vi "Save-Defaults.vi"(8 "error in (no error)":errorcluster, 9 "VI path":path, 11 "configuration file path":path) -> (0 "error out":errorcluster)   [LabVIEW 2020, in "Save-Load-Defaults.lvlib"]
doc: "This VI saves the controls of the VI specified in VI path to settings.dat using the Configuration File VIs."
uses:
  Save-Load-Defaults.lvlib
  <vilib>/Utility/config.llb/Write Key (String).vi
  <vilib>/Utility/config.llb/NI_LVConfig.lvlib
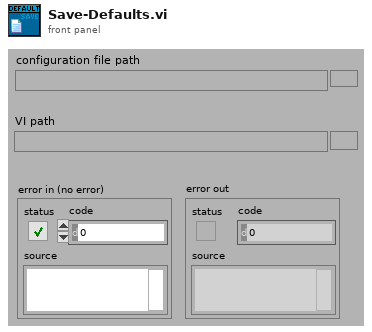
[diagram p1: front panel]
types:
  T1 = typedef "NI_LVConfig.lvlib/Config Data RefNum.ctl" = refnum<k1>
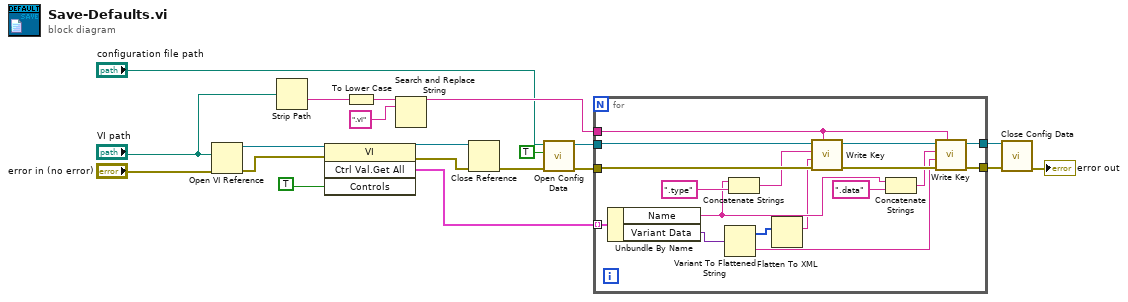
[diagram p0: block diagram]
diagram:
  n1 = Open VI Reference(vi path="VI path", error in (no error)="error in (no error)") -> (vi reference=w4:refnum<vi>, error out=w6:errorcluster)  [unwired: 4 in]
  n2 = Strip Path(path="VI path") -> (name=w19:string)  [unwired: 1 out]
  n3 = invoke class="VI" method="Ctrl Val.Get All"(reference=w4, error in=w6, "Controls"=TRUE ("controls")) -> (reference out=w8:refnum<vi>, error out=w9:errorcluster, "Get All Control Values Variant"=w7:cluster{"Name":string, "Variant Data":variant}[])  [unwired: 1 in, 1 out]
  n4 = To Lower Case(string=w19) -> (all lower case string=w20:string)
  n5 = Search and Replace String(input string=w20, search string=".vi") -> (result string=w18:string)  [unwired: 6 in, 3 out]
  n6 = Close Reference(reference=w8, error in (no error)=w9) -> (error out=w14:errorcluster)
  n7 = call <vilib>:"Open Config Data.vi"("error in (no error)"=w14, "create file if necessary (T)"=TRUE, "configuration file path"="configuration file path") -> ("error out"=w11:errorcluster, "refnum"=w10:T1)  [unwired: 6 in, 1 out]
  n8 = for {
    tunnel: w7 -> [w37] mode=indexing
    tunnel: w18 -> [w28]
    tunnel: w10 -> [w36]
    tunnel: w11 -> [w35]
    tunnel: [w27] -> w12
    tunnel: [w26] -> w13
    n9 = Unbundle By Name(w37) -> ("Name"=w25:string, "Variant Data"=w24:variant)
    n10 = Variant To Flattened String(Variant=w24) -> (data string=w21:string, 1:w23:i16[])
    n11 = Concatenate Strings(w25, ".type" ("string")) -> (w32:string)
    n12 = Flatten To XML(6:w23) -> (2:w22:string)
    n13 = call-poly <vilib>:"Write Key.vi"("section"=w28, "error in (no error)"=w35, "value"=w22, "key"=w32, "refnum"=w36) -> ("error out"=w30:errorcluster, "refnum out"=w31:T1)  [unwired: 4 in, 1 out]
    n14 = Concatenate Strings(w25, ".data" ("string")) -> (w29:string)
    n15 = call-poly <vilib>:"Write Key.vi"("section"=w28, "error in (no error)"=w30, "value"=w21, "key"=w29, "refnum"=w31) -> ("error out"=w26:errorcluster, "refnum out"=w27:T1)  [unwired: 4 in, 1 out]
  }
  n16 = call <vilib>:"Close Config Data.vi"("error in (no error)"=w13, "refnum"=w12) -> ("error out"=→"error out":errorcluster)  [unwired: 8 in, 1 out]
